vi "background3.vi"() -> ()   [LabVIEW 2014]
uses:
  cloud.ctl
  heart.ctl
  <vilib>/Utility/inputDevices.llb/keyboardAcquire.vi
  <vilib>/Utility/inputDevices.llb/closeKeyboard.vi
panel:
  out "Position:Top 3":i32
  out "Position:Left 3":i32
  out "人1生命":dbl
  out "人2生命":dbl
  out "heart 6":T1
  out "heart 5":T1
  out "heart 4":T1
  out "heart 3":T1
  out "heart 2":T1
  out "heart 1":T1
  out "雲  3":T2
  out "black hole":T3
  out "雲 2":T2
  out "雲":T2
  out "1jump":bool=TRUE
  out "火右飛 2":bool=TRUE
  out "火左飛 2":bool
  out "火左飛":bool
  out "1":T4
  out "火右飛":bool=TRUE
  out "2":T5
  out "2-1":T4
  out "2-2":T5
  in  "stop jump2":bool
  out "Position:Top 2":i32
  out "Position:Left 2":i32
  in  "stop jump1":bool
  out "人1":T6
  out "keys pressed":T7(array[ring])
  in  "right/left 2":bool
  in  "人2":bool
  in  "right/left":bool
  in  "人1":bool
  out "人2":T6
  out "Position:Top":i32
  out "Position:Left":i32
  in  "整個遊戲中止":bool
  # "W:17\nS:31\nA:30\nD:32"
  # "上:72\n下:80\n左:75\n右:77"
  # "17"
  # "48"
  # "587"
  # "168"
  # "523"
  # "623"
  # "678"
  # "334"
  # "288"
  # "408"
  # "1049"
  # "212"
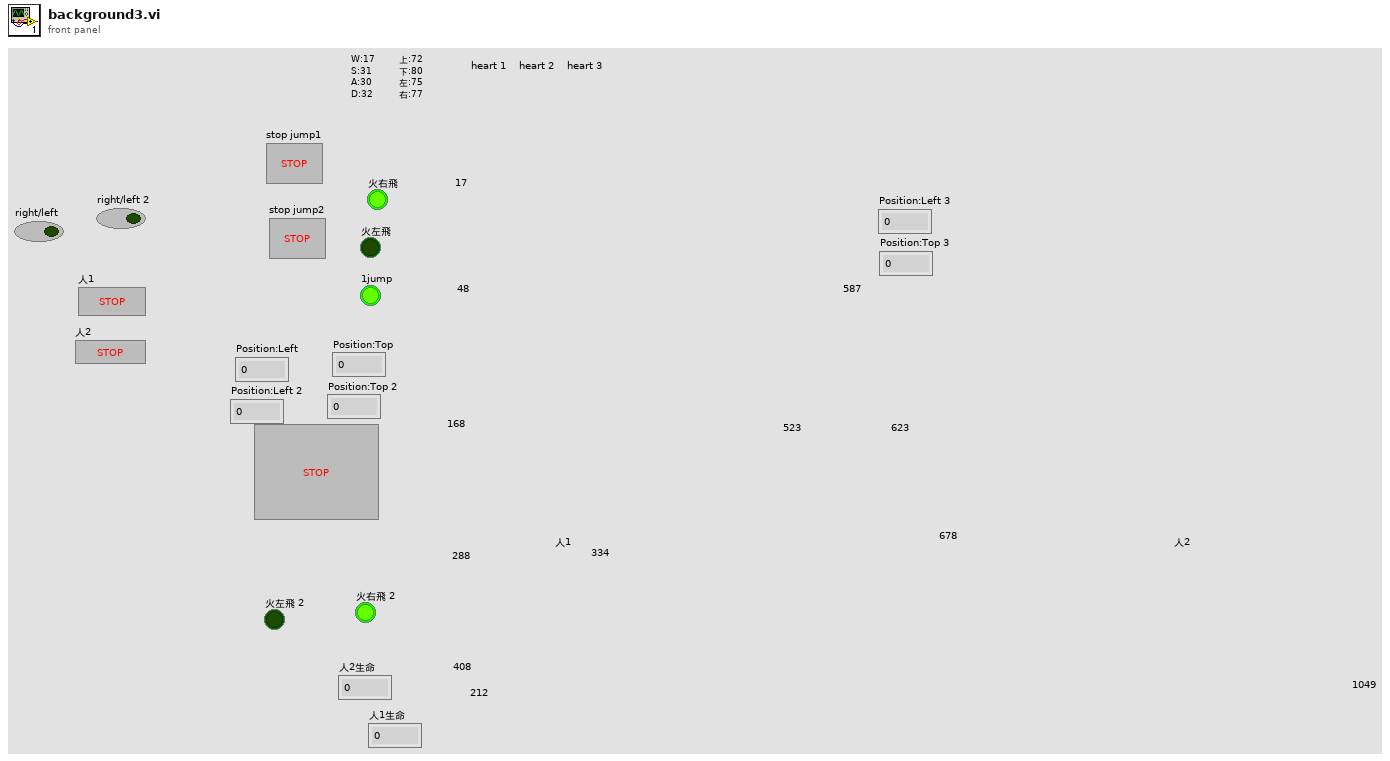
[diagram p1: front panel]
types:
  T1 = typedef "heart.ctl" = u16
  T2 = typedef "cloud.ctl" = u16
  T3 = typedef "Control 4.ctl" = u16
  T4 = typedef "火焰.ctl" = u16
  T5 = typedef "火焰2.ctl" = u16
  T6 = typedef "Control 3.ctl" = u16
  T7 = enum16{"0", "1", "2", "3", "4", "5", "6", "7", "8", "9", "A", "B", "C", "D", "E", "F", "G", "H", "I", "J", "K", "L", "M", "N", "O", "P", "Q", "R", "S", "T", "U", "V", "W", "X", "Y", "Z", "F1", "F2", "F3", "F4", "F5", "F6", "F7", "F8", "F9", "F10", "F11", "F12", "F13", "F14", "F15", "ADD", "BACK", "BACKSLASH", "CAPITAL", "COMMA", "DECIMAL", "DELETE", "DIVIDE", "DOWN", "END", "EQUALS", "ESCAPE", "GRAVE (`)", "HOME", "INSERT", "LBRACKET", "LCONTROL", "LEFT", "L ALT", "LSHIFT", "LWIN", "MINUS", "MULTIPLY", "NEXT", "NUMLOCK", "NUMPAD_0", "NUMPAD_1", "NUMPAD_2", "NUMPAD_3", "NUMPAD_4", "NUMPAD_5", "NUMPAD_6", "NUMPAD_7", "NUMPAD_8", "NUMPAD_9", "PAUSE", "PERIOD", "PRIOR (PG UP)", "RBRACKET", "RCONTROL", "RETURN", "RIGHT", "R ALT", "RSHIFT", "RWIN", "SCROLL", "SEMICOLON", "SLASH", "SPACE", "SUBTRACT", "TAB", "UP", "ENTER (num pad)", "' (quote)"}[]
  T8 = enum16{"0", "1", "2", "3", "4", "5", "6", "7", "8", "9", "A", "B", "C", "D", "E", "F", "G", "H", "I", "J", "K", "L", "M", "N", "O", "P", "Q", "R", "S", "T", "U", "V", "W", "X", "Y", "Z", "F1", "F2", "F3", "F4", "F5", "F6", "F7", "F8", "F9", "F10", "F11", "F12", "F13", "F14", "F15", "ADD", "BACK", "BACKSLASH", "CAPITAL", "COMMA", "DECIMAL", "DELETE", "DIVIDE", "DOWN", "END", "EQUALS", "ESCAPE", "GRAVE (`)", "HOME", "INSERT", "LBRACKET", "LCONTROL", "LEFT", "L ALT", "LSHIFT", "LWIN", "MINUS", "MULTIPLY", "NEXT", "NUMLOCK", "NUMPAD_0", "NUMPAD_1", "NUMPAD_2", "NUMPAD_3", "NUMPAD_4", "NUMPAD_5", "NUMPAD_6", "NUMPAD_7", "NUMPAD_8", "NUMPAD_9", "PAUSE", "PERIOD", "PRIOR (PG UP)", "RBRACKET", "RCONTROL", "RETURN", "RIGHT", "R ALT", "RSHIFT", "RWIN", "SCROLL", "SEMICOLON", "SLASH", "SPACE", "SUBTRACT", "TAB", "UP", "ENTER (num pad)", "' (quote)"}
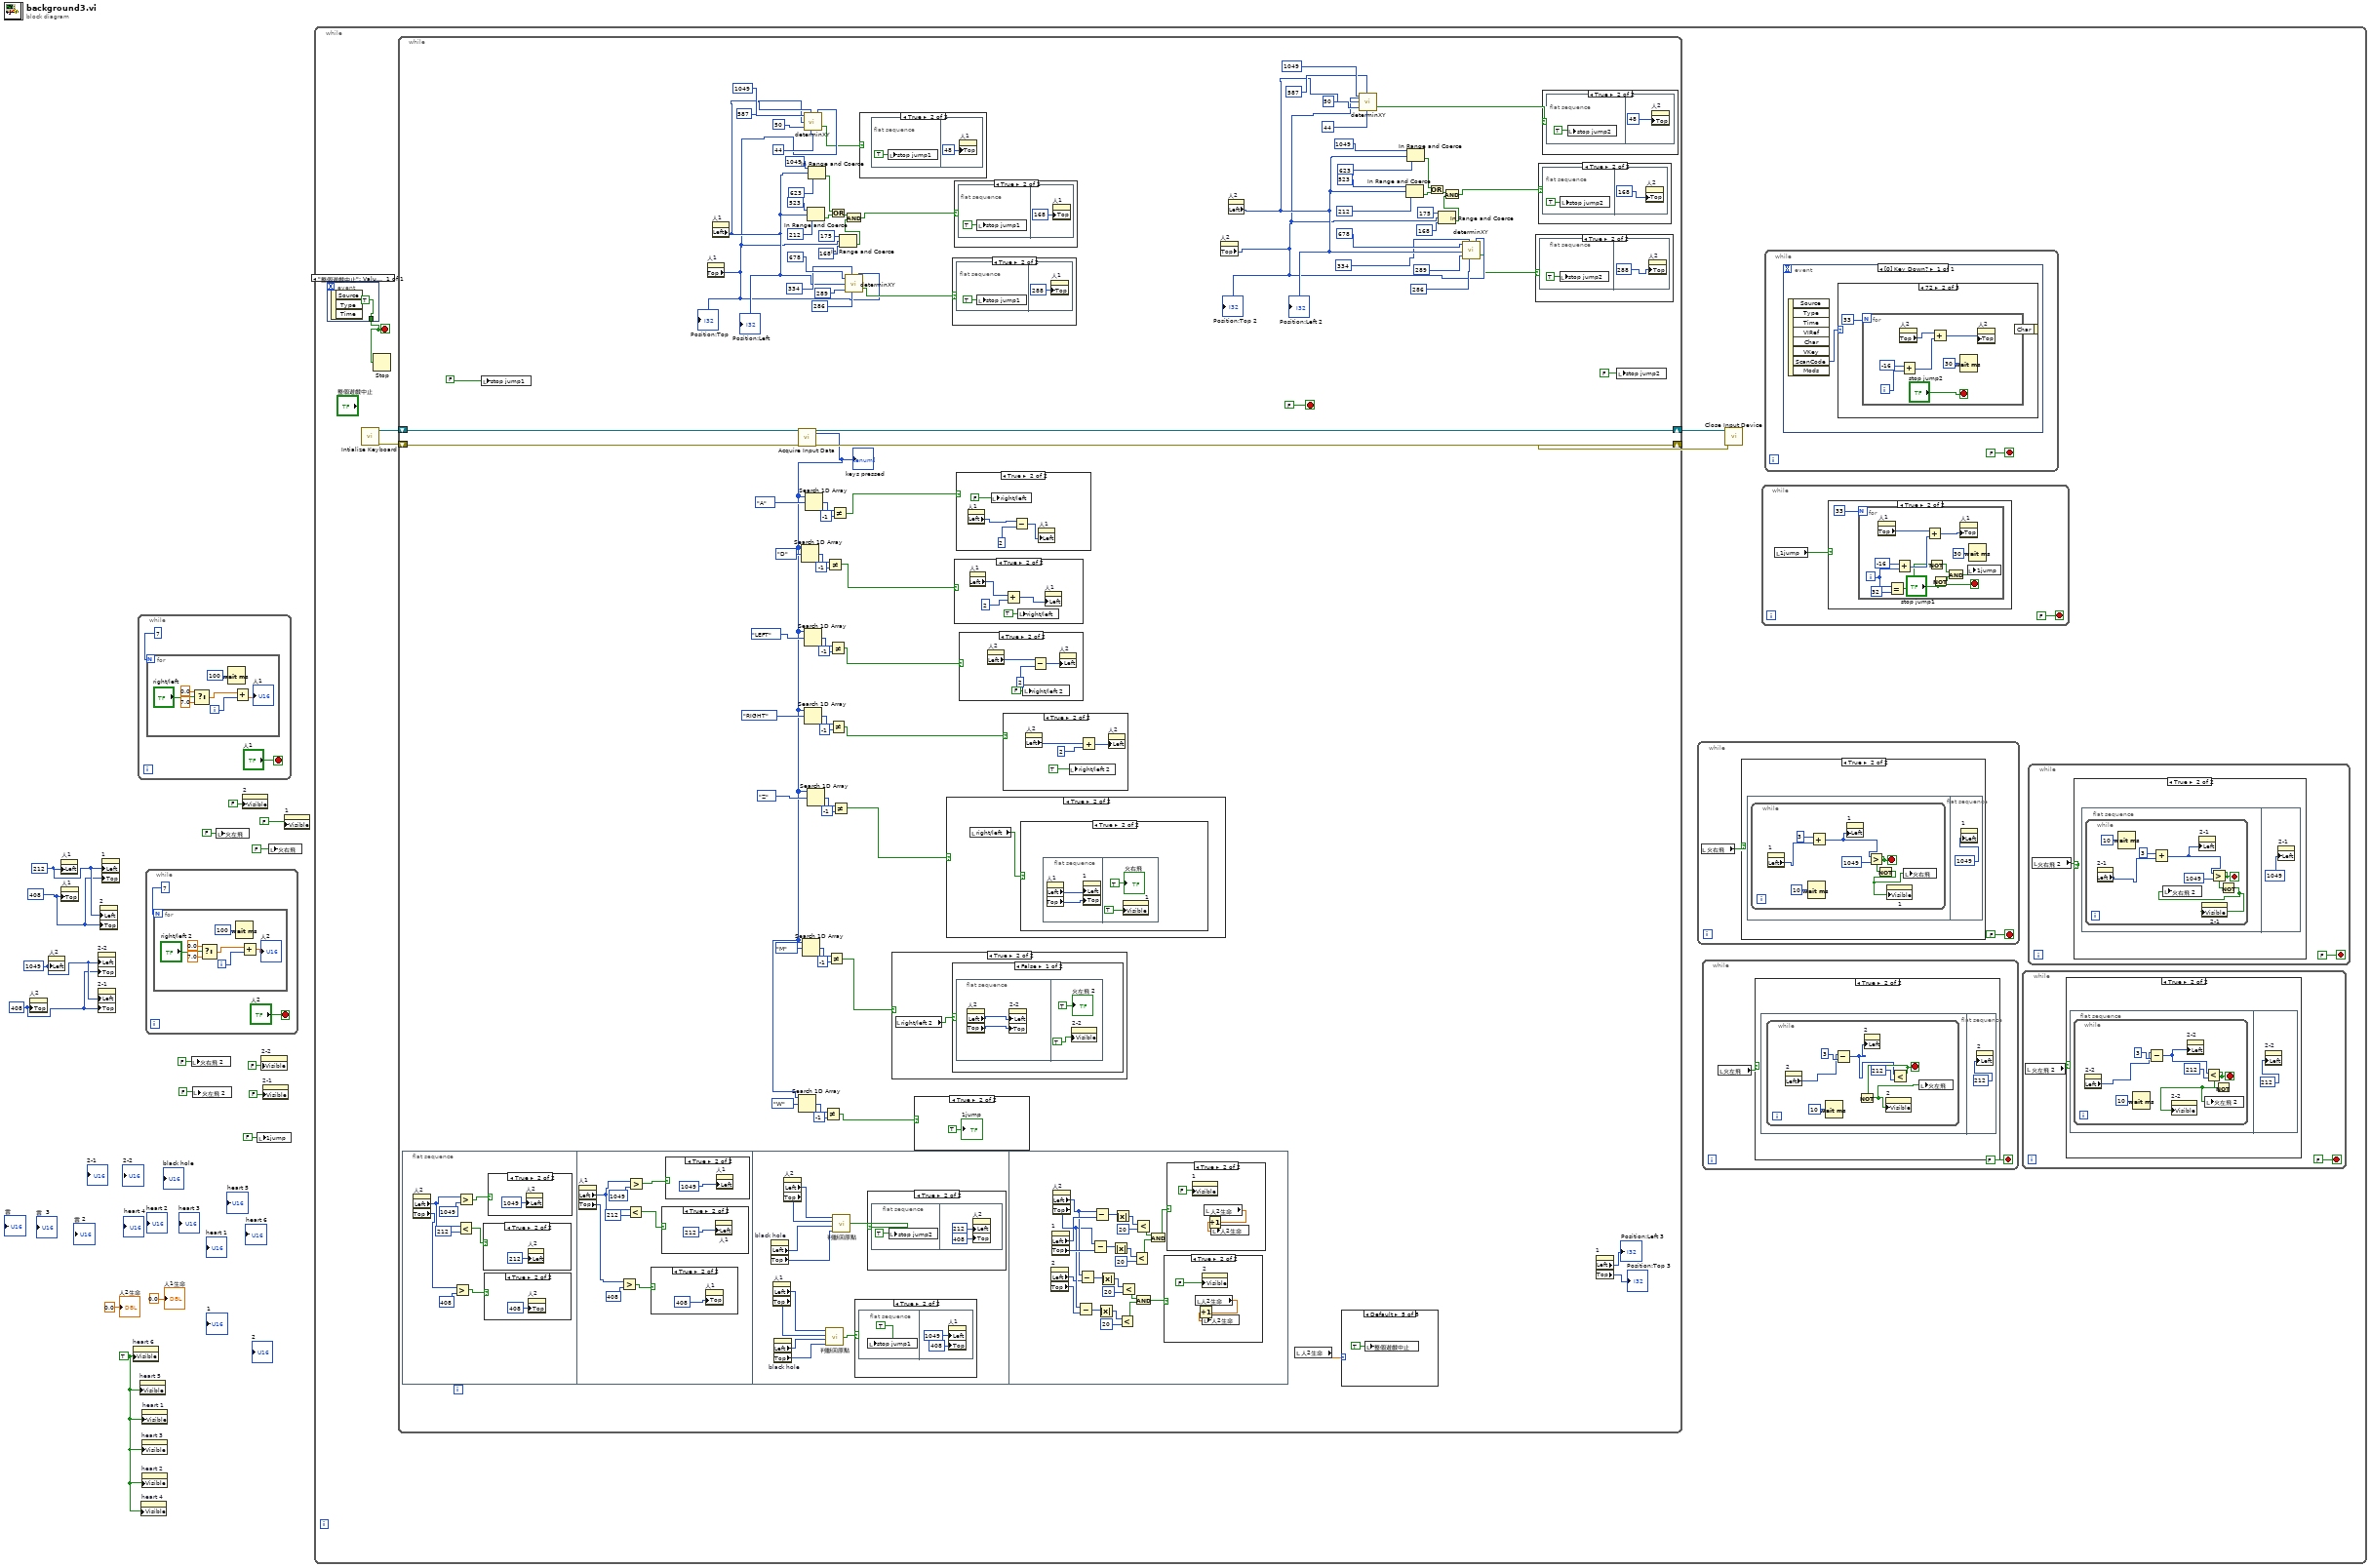
[diagram p0: block diagram]
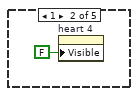
[diagram p10: hidden frame]
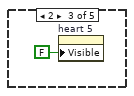
[diagram p11: hidden frame]
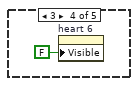
[diagram p12: hidden frame]
diagram:
  w1 = TRUE ("Visible")
  w5 = 408 ("Position:Top")
  w6 = 1049 ("Position:Left")
  w7 = 408 ("Position:Top")
  w8 = 212 ("Position:Left")
  n1 = property on="人2" class="Ring (strict)"("Top"=w5) -> ()  [unwired: 2 in, 2 out]
  n2 = property on="人2" class="Ring (strict)"("Left"=w6) -> ()  [unwired: 2 in, 2 out]
  n3 = property on="人1" class="Ring (strict)"("Left"=w8) -> ()  [unwired: 2 in, 2 out]
  n4 = property on="人1" class="Ring (strict)"("Top"=w7) -> ()  [unwired: 2 in, 2 out]
  n5 = property on="2-2" class="Ring (strict)"("Left"=w6, "Top"=w5) -> ()  [unwired: 2 in, 2 out]
  n6 = property on="2-1" class="Ring (strict)"("Left"=w6, "Top"=w5) -> ()  [unwired: 2 in, 2 out]
  n7 = property on="2" class="Ring (strict)"("Left"=w8, "Top"=w7) -> ()  [unwired: 2 in, 2 out]
  n8 = property on="1" class="Ring (strict)"("Left"=w8, "Top"=w7) -> ()  [unwired: 2 in, 2 out]
  n9 = property on="heart 6" class="Ring (strict)"("Visible"=w1) -> ()  [unwired: 2 in, 2 out]
  n10 = while {
    stop <- "人1" stop-if-true
    n11 = for {
      N: 7 -> [_]
      i -> [w24]
      n12 = Select(t=0.0, s="right/left", f=7.0) -> (s? t:f=w21:dbl)
      n13 = Wait (ms)(milliseconds to wait=u32 100) -> ()  [unwired: 1 out]
      n14 = Add(x=w21, y=w24) -> (x+y=→"人1":dbl)
    }
  }
  n15 = property on="heart 5" class="Ring (strict)"("Visible"=w1) -> ()  [unwired: 2 in, 2 out]
  n16 = property on="heart 4" class="Ring (strict)"("Visible"=w1) -> ()  [unwired: 2 in, 2 out]
  n17 = property on="heart 3" class="Ring (strict)"("Visible"=w1) -> ()  [unwired: 2 in, 2 out]
  n18 = property on="heart 2" class="Ring (strict)"("Visible"=w1) -> ()  [unwired: 2 in, 2 out]
  n19 = property on="heart 1" class="Ring (strict)"("Visible"=w1) -> ()  [unwired: 2 in, 2 out]
  n20 = while {
    stop <- "人2" stop-if-true
    n21 = for {
      N: 7 -> [_]
      i -> [w33]
      n22 = Select(t=0.0, s="right/left 2", f=7.0) -> (s? t:f=w31:dbl)
      n23 = Wait (ms)(milliseconds to wait=u32 100) -> ()  [unwired: 1 out]
      n24 = Add(x=w31, y=w33) -> (x+y=→"人2":dbl)
    }
  }
  n25 = local write "火右飛 2"(FALSE ("火右飛 2")) -> ()
  n26 = local write "火左飛 2"(FALSE ("火左飛 2")) -> ()
  n27 = local write "火左飛"(FALSE ("火左飛")) -> ()
  n28 = property on="2" class="Ring (strict)"("Visible"=FALSE) -> ()  [unwired: 2 in, 2 out]
  n29 = local write "1jump"(FALSE ("1jump")) -> ()
  n30 = property on="2-2" class="Ring (strict)"("Visible"=FALSE) -> ()  [unwired: 2 in, 2 out]
  n31 = property on="2-1" class="Ring (strict)"("Visible"=FALSE) -> ()  [unwired: 2 in, 2 out]
  n32 = local write "火右飛"(FALSE ("Boolean")) -> ()
  n33 = property on="1" class="Ring (strict)"("Visible"=FALSE) -> ()  [unwired: 2 in, 2 out]
  n34 = while {
    stop <- w35 stop-if-true
    n35 = event shown="[0] \"整個遊戲中止\": Value Change" {
      selector: _ -> [_]
      dyn-events: _ -> [_]
      timeout: _ -> [_]
      tunnel: [TRUE] -> w35
      event "整個遊戲中止": Value Change {
        n36 = event-data() -> ()  [unwired: 1 in, 3 out]
      }
    }
    n37 = call <vilib>:"Intialize Keyboard.vi"() -> ("error out"=w38:errorcluster, "device ID"=w39:refnum<k1>)  [unwired: 10 in]
    n38 = Stop(stop? (T)=w35) -> ()
    n39 = while {
      shift-right: [w190] -> w36
      shift-left: w39 -> [w187]
      shift-right: [w189] -> w37
      shift-left: w38 -> [w188]
      stop <- FALSE stop-if-true
      n40 = flat-sequence {
        frame #0 {
          n41 = property on="人2" class="Ring (strict)"() -> ("Left"=w201:i32, "Top"=w196:i32)  [unwired: 2 in, 2 out]
          n42 = Greater?(x=w196, y=408) -> (0:w195:bool)
          n43 = Less?(x=w201, y=212) -> (x < y?=w198:bool)
          n44 = Greater?(x=w201, y=1049) -> (0:w199:bool)
          n45 = case shown="True" w198 {
            frame False {
            }
            frame True {
              n46 = property on="人2" class="Ring (strict)"("Left"=212 ("Position:Left")) -> ()  [unwired: 2 in, 2 out]
            }
          }
          n47 = case shown="True" w195 {
            frame False {
            }
            frame True {
              n48 = property on="人2" class="Ring (strict)"("Top"=408 ("Position:Left")) -> ()  [unwired: 2 in, 2 out]
            }
          }
          n49 = case shown="True" w199 {
            frame False {
            }
            frame True {
              n50 = property on="人2" class="Ring (strict)"("Left"=1049 ("Position:Left")) -> ()  [unwired: 2 in, 2 out]
            }
          }
        }
        frame #1 {
          n51 = property on="人1" class="Ring (strict)"() -> ("Left"=w213:i32, "Top"=w206:i32)  [unwired: 2 in, 2 out]
          n52 = Greater?(x=w206, y=408) -> (0:w208:bool)
          n53 = Less?(x=w213, y=212) -> (x < y?=w212:bool)
          n54 = Greater?(x=w213, y=1049) -> (0:w211:bool)
          n55 = case shown="True" w208 {
            frame False {
            }
            frame True {
              n56 = property on="人1" class="Ring (strict)"("Top"=408 ("Position:Left")) -> ()  [unwired: 2 in, 2 out]
            }
          }
          n57 = case shown="True" w212 {
            frame False {
            }
            frame True {
              n58 = property on="人1" class="Ring (strict)"("Left"=212 ("Position:Left")) -> ()  [unwired: 2 in, 2 out]
            }
          }
          n59 = case shown="True" w211 {
            frame False {
            }
            frame True {
              n60 = property on="人1" class="Ring (strict)"("Left"=1049 ("Position:Left")) -> ()  [unwired: 2 in, 2 out]
            }
          }
        }
        frame #2 {
          n61 = property on="black hole" class="Ring (strict)"() -> ("Left"=w224:i32, "Top"=w223:i32)  [unwired: 2 in, 2 out]
          n62 = property on="人1" class="Ring (strict)"() -> ("Left"=w217:i32, "Top"=w218:i32)  [unwired: 2 in, 2 out]
          n63 = property on="black hole" class="Ring (strict)"() -> ("Left"=w219:i32, "Top"=w220:i32)  [unwired: 2 in, 2 out]
          n64 = property on="人2" class="Ring (strict)"() -> ("Left"=w226:i32, "Top"=w225:i32)  [unwired: 2 in, 2 out]
          n65 = call "判斷回原點.vi"("¬}y"=w220, "¬}x"=w219, "人y"=w218, "人x"=w217) -> ("x .and. y?"=w221:bool)
          n66 = call "判斷回原點.vi"("¬}y"=w223, "¬}x"=w224, "人y"=w225, "人x"=w226) -> ("x .and. y?"=w222:bool)
          n67 = case shown="True" w221 {
            frame False {
            }
            frame True {
              n68 = flat-sequence {
                frame #0 {
                  n69 = local write "stop jump1"(TRUE) -> ()
                }
                frame #1 {
                  n70 = property on="人1" class="Ring (strict)"("Left"=1049 ("Position:Left"), "Top"=408 ("Position:Top")) -> ()  [unwired: 2 in, 2 out]
                }
              }
            }
          }
          n71 = case shown="True" w222 {
            frame False {
            }
            frame True {
              n72 = flat-sequence {
                frame #0 {
                  n73 = local write "stop jump2"(TRUE ("stop jump2")) -> ()
                }
                frame #1 {
                  n74 = property on="人2" class="Ring (strict)"("Left"=212 ("Position:Left"), "Top"=408 ("Position:Top")) -> ()  [unwired: 2 in, 2 out]
                }
              }
            }
          }
        }
        frame #3 {
          n75 = property on="2" class="Ring (strict)"() -> ("Left"=w234:i32, "Top"=w233:i32)  [unwired: 2 in, 2 out]
          n76 = property on="1" class="Ring (strict)"() -> ("Left"=w256:i32, "Top"=w249:i32)  [unwired: 2 in, 2 out]
          n77 = property on="人2" class="Ring (strict)"() -> ("Left"=w236:i32, "Top"=w235:i32)  [unwired: 2 in, 2 out]
          n78 = Subtract(x=w235, y=w233) -> (x-y=w243:i32)
          n79 = Subtract(x=w236, y=w234) -> (x-y=w238:i32)
          n80 = Subtract(x=w235, y=w249) -> (x-y=w250:i32)
          n81 = Subtract(x=w236, y=w256) -> (x-y=w255:i32)
          n82 = Absolute Value(x=w243) -> (abs(x)=w242:i32)
          n83 = Absolute Value(x=w238) -> (abs(x)=w239:i32)
          n84 = Absolute Value(x=w250) -> (abs(x)=w251:i32)
          n85 = Absolute Value(x=w255) -> (abs(x)=w254:i32)
          n86 = Less?(x=w242, y=20) -> (x < y?=w245:bool)
          n87 = Less?(x=w239, y=20) -> (x < y?=w244:bool)
          n88 = Less?(x=w251, y=20) -> (x < y?=w247:bool)
          n89 = Less?(x=w254, y=20) -> (x < y?=w248:bool)
          n90 = And(x=w244, y=w245) -> (x .and. y?=w237:bool)
          n91 = And(x=w248, y=w247) -> (x .and. y?=w246:bool)
          n92 = case shown="True" w237 {
            frame False {
            }
            frame True {
              n93 = local read "人2生命"() -> (w257:dbl)
              n94 = Increment(x=w257) -> (x+1=w258:dbl)
              n95 = property on="2" class="Ring (strict)"("Visible"=FALSE) -> ()  [unwired: 2 in, 2 out]
              n96 = local write "人2生命"(w258) -> ()
            }
          }
          n97 = case shown="True" w246 {
            frame False {
            }
            frame True {
              n98 = property on="1" class="Ring (strict)"("Visible"=FALSE) -> ()  [unwired: 2 in, 2 out]
              n99 = local read "人2生命"() -> (w261:dbl)
              n100 = Increment(x=w261) -> (x+1=w260:dbl)
              n101 = local write "人2生命"(w260) -> ()
            }
          }
        }
      }
      n102 = local write "stop jump1"(FALSE ("stop jump1")) -> ()
      n103 = property on="人1" class="Ring (strict)"() -> ("Top"=w122:i32)  [unwired: 2 in, 2 out]
      "Position:Top" <- w122
      n104 = property on="人1" class="Ring (strict)"() -> ("Left"=w125:i32)  [unwired: 2 in, 2 out]
      "Position:Left" <- w125
      n105 = call-poly <vilib>:"Acquire Input Data.vi"("device ID"=w187, "error in (no error)"=w188) -> ("device ID"=w190:refnum<k1>, "keys pressed"=w134:T7, "error out"=w189:errorcluster)  [unwired: 15 in]
      "keys pressed" <- w134
      n106 = Search 1D Array(1D array=w134, element=T8."W") -> (index of element=w136:i32)  [unwired: 1 in]
      n107 = Search 1D Array(1D array=w134, element=T8."D") -> (index of element=w181:i32)  [unwired: 1 in]
      n108 = Search 1D Array(1D array=w134, element=T8."M") -> (index of element=w143:i32)  [unwired: 1 in]
      n109 = call "determinXY.vi"("x max"=1049 ("upper limit"), "x min"=587 ("lower limit"), "x"=w125, "y max"=50 ("upper limit"), "y min"=44 ("lower limit"), "y"=w122) -> ("result"=w121:bool)
      n110 = Search 1D Array(1D array=w134, element=T8."LEFT") -> (index of element=w178:i32)  [unwired: 1 in]
      n111 = Search 1D Array(1D array=w134, element=T8."RIGHT") -> (index of element=w174:i32)  [unwired: 1 in]
      n112 = Search 1D Array(1D array=w134, element=T8."A") -> (index of element=w184:i32)  [unwired: 1 in]
      n113 = Search 1D Array(1D array=w134, element=T8."Z") -> (index of element=w146:i32)  [unwired: 1 in]
      n114 = In Range and Coerce(upper limit=523, x=w125, lower limit=212) -> (In Range?=w161:bool)  [unwired: 1 out]
      n115 = In Range and Coerce(upper limit=1049, x=w125, lower limit=623) -> (In Range?=w162:bool)  [unwired: 1 out]
      n116 = Not Equal?(x=w136, y=-1) -> (x != y?=w133:bool)
      n117 = Not Equal?(x=w181, y=-1) -> (x != y?=w139:bool)
      n118 = Not Equal?(x=w143, y=-1) -> (x != y?=w141:bool)
      n119 = Not Equal?(x=w178, y=-1) -> (x != y?=w176:bool)
      n120 = Or(x=w162, y=w161) -> (x .or. y?=w163:bool)
      n121 = Not Equal?(x=w174, y=-1) -> (x != y?=w172:bool)
      n122 = Not Equal?(x=w184, y=-1) -> (x != y?=w140:bool)
      n123 = Not Equal?(x=w146, y=-1) -> (x != y?=w138:bool)
      n124 = In Range and Coerce(upper limit=175, x=w122, lower limit=168 ("y")) -> (In Range?=w167:bool)  [unwired: 1 out]
      n125 = And(x=w163, y=w167) -> (x .and. y?=w160:bool)
      n126 = call "determinXY.vi"("x max"=678 ("upper limit"), "x min"=334 ("lower limit"), "x"=w125, "y max"=289 ("upper limit"), "y min"=286 ("y"), "y"=w122) -> ("result"=w128:bool)
      n127 = case shown="True" w121 {
        frame False {
        }
        frame True {
          n128 = flat-sequence {
            frame #0 {
              n129 = local write "stop jump1"(TRUE ("stop jump1")) -> ()
            }
            frame #1 {
              n130 = property on="人1" class="Ring (strict)"("Top"=48 ("Position:Top")) -> ()  [unwired: 2 in, 2 out]
            }
          }
        }
      }
      n131 = case shown="True" w141 {
        frame False {
        }
        frame True {
          n132 = local read "right/left 2"() -> (w264:bool)
          n133 = case shown="False" w264 {
            frame False {
              n134 = flat-sequence {
                frame #0 {
                  n135 = property on="人2" class="Ring (strict)"() -> ("Left"=w266:i32, "Top"=w265:i32)  [unwired: 2 in, 2 out]
                  n136 = property on="2-2" class="Ring (strict)"("Left"=w266, "Top"=w265) -> ()  [unwired: 2 in, 2 out]
                }
                frame #1 {
                  n137 = property on="2-2" class="Ring (strict)"("Visible"=TRUE) -> ()  [unwired: 2 in, 2 out]
                  "火左飛 2" <- TRUE
                }
              }
            }
            frame True {
              n138 = flat-sequence {
                frame #0 {
                  n139 = property on="人2" class="Ring (strict)"() -> ("Left"=w270:i32, "Top"=w269:i32)  [unwired: 2 in, 2 out]
                  n140 = property on="2-1" class="Ring (strict)"("Left"=w270, "Top"=w269) -> ()  [unwired: 2 in, 2 out]
                }
                frame #1 {
                  n141 = property on="2-1" class="Ring (strict)"("Visible"=TRUE) -> ()  [unwired: 2 in, 2 out]
                  "火右飛 2" <- TRUE
                }
              }
            }
          }
        }
      }
      n142 = case shown="True" w133 {
        frame False {
        }
        frame True {
          "1jump" <- TRUE
        }
      }
      n143 = case shown="True" w138 {
        frame False {
        }
        frame True {
          n144 = local read "right/left"() -> (w273:bool)
          n145 = case shown="True" w273 {
            frame False {
              n146 = flat-sequence {
                frame #0 {
                  n147 = property on="人1" class="Ring (strict)"() -> ("Left"=w275:i32, "Top"=w274:i32)  [unwired: 2 in, 2 out]
                  n148 = property on="2" class="Ring (strict)"("Left"=w275, "Top"=w274) -> ()  [unwired: 2 in, 2 out]
                }
                frame #1 {
                  n149 = property on="2" class="Ring (strict)"("Visible"=TRUE) -> ()  [unwired: 2 in, 2 out]
                  "火左飛" <- TRUE
                }
              }
            }
            frame True {
              n150 = flat-sequence {
                frame #0 {
                  n151 = property on="人1" class="Ring (strict)"() -> ("Left"=w279:i32, "Top"=w278:i32)  [unwired: 2 in, 2 out]
                  n152 = property on="1" class="Ring (strict)"("Left"=w279, "Top"=w278) -> ()  [unwired: 2 in, 2 out]
                }
                frame #1 {
                  n153 = property on="1" class="Ring (strict)"("Visible"=TRUE) -> ()  [unwired: 2 in, 2 out]
                  "火右飛" <- TRUE
                }
              }
            }
          }
        }
      }
      n154 = case shown="True" w128 {
        frame False {
        }
        frame True {
          n155 = flat-sequence {
            frame #0 {
              n156 = local write "stop jump1"(TRUE ("stop jump1")) -> ()
            }
            frame #1 {
              n157 = property on="人1" class="Ring (strict)"("Top"=288 ("Position:Top")) -> ()  [unwired: 2 in, 2 out]
            }
          }
        }
      }
      n158 = case shown="True" w160 {
        frame False {
        }
        frame True {
          n159 = flat-sequence {
            frame #0 {
              n160 = local write "stop jump1"(TRUE ("stop jump1")) -> ()
            }
            frame #1 {
              n161 = property on="人1" class="Ring (strict)"("Top"=168 ("Position:Top")) -> ()  [unwired: 2 in, 2 out]
            }
          }
        }
      }
      n162 = case shown="True" w139 {
        frame False {
        }
        frame True {
          n163 = property on="人1" class="Ring (strict)"() -> ("Left"=w304:i32)  [unwired: 2 in, 2 out]
          n164 = Add(x=w304, y=2) -> (x+y=w303:i32)
          n165 = local write "right/left"(TRUE ("right/left")) -> ()
          n166 = property on="人1" class="Ring (strict)"("Left"=w303) -> ()  [unwired: 2 in, 2 out]
        }
      }
      n167 = case shown="True" w140 {
        frame False {
        }
        frame True {
          n168 = property on="人1" class="Ring (strict)"() -> ("Left"=w307:i32)  [unwired: 2 in, 2 out]
          n169 = local write "right/left"(FALSE ("人1 right 2")) -> ()
          n170 = Subtract(x=w307, y=2) -> (x-y=w306:i32)
          n171 = property on="人1" class="Ring (strict)"("Left"=w306) -> ()  [unwired: 2 in, 2 out]
        }
      }
      n172 = case shown="True" w176 {
        frame False {
        }
        frame True {
          n173 = property on="人2" class="Ring (strict)"() -> ("Left"=w300:i32)  [unwired: 2 in, 2 out]
          n174 = local write "right/left 2"(FALSE ("right/left")) -> ()
          n175 = Subtract(x=w300, y=2) -> (x-y=w299:i32)
          n176 = property on="人2" class="Ring (strict)"("Left"=w299) -> ()  [unwired: 2 in, 2 out]
        }
      }
      n177 = case shown="True" w172 {
        frame False {
        }
        frame True {
          n178 = property on="人2" class="Ring (strict)"() -> ("Left"=w296:i32)  [unwired: 2 in, 2 out]
          n179 = local write "right/left 2"(TRUE ("人1 right 2")) -> ()
          n180 = Add(x=w296, y=2) -> (x+y=w295:i32)
          n181 = property on="人2" class="Ring (strict)"("Left"=w295) -> ()  [unwired: 2 in, 2 out]
        }
      }
      n182 = property on="人2" class="Ring (strict)"() -> ("Top"=w110:i32)  [unwired: 2 in, 2 out]
      "Position:Top 2" <- w110
      n183 = property on="人2" class="Ring (strict)"() -> ("Left"=w114:i32)  [unwired: 2 in, 2 out]
      "Position:Left 2" <- w114
      n184 = local read "人2生命"() -> (w106:dbl)
      n185 = case shown="Default" w106 {
        frame 0 {
        }
        frame 1 {
          n186 = property on="heart 4" class="Ring (strict)"("Visible"=FALSE) -> ()  [unwired: 2 in, 2 out]
        }
        frame 2 {
          n187 = property on="heart 5" class="Ring (strict)"("Visible"=FALSE) -> ()  [unwired: 2 in, 2 out]
        }
        frame 3 {
          n188 = property on="heart 6" class="Ring (strict)"("Visible"=FALSE) -> ()  [unwired: 2 in, 2 out]
        }
        frame Default {
          n189 = local write "整個遊戲中止"(TRUE ("整個遊戲中止")) -> ()
        }
      }
      n190 = call "determinXY.vi"("x max"=1049 ("upper limit"), "x min"=587 ("lower limit"), "x"=w114, "y max"=50 ("upper limit"), "y min"=44 ("lower limit"), "y"=w110) -> ("result"=w116:bool)
      n191 = In Range and Coerce(upper limit=523, x=w114, lower limit=212) -> (In Range?=w150:bool)  [unwired: 1 out]
      n192 = In Range and Coerce(upper limit=1049, x=w114, lower limit=623) -> (In Range?=w151:bool)  [unwired: 1 out]
      n193 = Or(x=w151, y=w150) -> (x .or. y?=w152:bool)
      n194 = In Range and Coerce(upper limit=175, x=w110, lower limit=168 ("y")) -> (In Range?=w155:bool)  [unwired: 1 out]
      n195 = And(x=w152, y=w155) -> (x .and. y?=w149:bool)
      n196 = call "determinXY.vi"("x max"=678 ("upper limit"), "x min"=334 ("lower limit"), "x"=w114, "y max"=289 ("upper limit"), "y min"=286 ("y"), "y"=w110) -> ("result"=w109:bool)
      n197 = case shown="True" w109 {
        frame False {
        }
        frame True {
          n198 = flat-sequence {
            frame #0 {
              n199 = local write "stop jump2"(TRUE ("stop jump1")) -> ()
            }
            frame #1 {
              n200 = property on="人2" class="Ring (strict)"("Top"=288 ("Position:Top")) -> ()  [unwired: 2 in, 2 out]
            }
          }
        }
      }
      n201 = case shown="True" w149 {
        frame False {
        }
        frame True {
          n202 = flat-sequence {
            frame #0 {
              n203 = local write "stop jump2"(TRUE ("stop jump1")) -> ()
            }
            frame #1 {
              n204 = property on="人2" class="Ring (strict)"("Top"=168 ("Position:Top")) -> ()  [unwired: 2 in, 2 out]
            }
          }
        }
      }
      n205 = case shown="True" w116 {
        frame False {
        }
        frame True {
          n206 = flat-sequence {
            frame #0 {
              n207 = local write "stop jump2"(TRUE ("stop jump1")) -> ()
            }
            frame #1 {
              n208 = property on="人2" class="Ring (strict)"("Top"=48 ("Position:Top")) -> ()  [unwired: 2 in, 2 out]
            }
          }
        }
      }
      n209 = property on="1" class="Ring (strict)"() -> ("Left"=→"Position:Left 3":i32, "Top"=→"Position:Top 3":i32)  [unwired: 2 in, 2 out]
      n210 = local write "stop jump2"(FALSE ("stop jump1 2")) -> ()
    }
    n211 = while {
      stop <- FALSE stop-if-true
      n212 = local read "火右飛"() -> (w77:bool)
      n213 = case shown="True" w77 {
        frame False {
        }
        frame True {
          n214 = flat-sequence {
            frame #0 {
              n215 = while {
                stop <- w82 stop-if-true
                n216 = property on="1" class="Ring (strict)"() -> ("Left"=w81:i32)  [unwired: 2 in, 2 out]
                n217 = Wait (ms)(milliseconds to wait=u32 10) -> ()  [unwired: 1 out]
                n218 = Add(x=3, y=w81) -> (x+y=w80:i32)
                n219 = property on="1" class="Ring (strict)"("Left"=w80) -> ()  [unwired: 2 in, 2 out]
                n220 = Greater?(x=w80, y=1049) -> (0:w82:bool)
                n221 = Not(x=w82) -> (.not. x?=w78:bool)
                n222 = property on="1" class="Ring (strict)"("Visible"=w78) -> ()  [unwired: 2 in, 2 out]
                n223 = local write "火右飛"(w78) -> ()
              }
            }
            frame #1 {
              n224 = property on="1" class="Ring (strict)"("Left"=1049 ("y")) -> ()  [unwired: 2 in, 2 out]
            }
          }
        }
      }
    }
    n225 = while {
      stop <- FALSE stop-if-true
      n226 = local read "火左飛"() -> (w87:bool)
      n227 = case shown="True" w87 {
        frame False {
        }
        frame True {
          n228 = flat-sequence {
            frame #0 {
              n229 = while {
                stop <- w94 stop-if-true
                n230 = property on="2" class="Ring (strict)"() -> ("Left"=w92:i32)  [unwired: 2 in, 2 out]
                n231 = Wait (ms)(milliseconds to wait=u32 10) -> ()  [unwired: 1 out]
                n232 = Subtract(x=w92, y=3 ("x")) -> (x-y=w89:i32)
                n233 = property on="2" class="Ring (strict)"("Left"=w89) -> ()  [unwired: 2 in, 2 out]
                n234 = Less?(x=w89, y=212) -> (x < y?=w94:bool)
                n235 = Not(x=w94) -> (.not. x?=w88:bool)
                n236 = property on="2" class="Ring (strict)"("Visible"=w88) -> ()  [unwired: 2 in, 2 out]
                n237 = local write "火左飛"(w88) -> ()
              }
            }
            frame #1 {
              n238 = property on="2" class="Ring (strict)"("Left"=212 ("y")) -> ()  [unwired: 2 in, 2 out]
            }
          }
        }
      }
    }
    n239 = call-poly <vilib>:"Close Input Device.vi"("error in (no error)"=w37, "device ID"=w36) -> ()  [unwired: 8 in, 1 out]
    n240 = while {
      stop <- FALSE stop-if-true
      n241 = local read "1jump"() -> (w41:bool)
      n242 = case shown="True" w41 {
        frame False {
        }
        frame True {
          n243 = for {
            N: 33 -> [_]
            i -> [w49]
            stop <- "stop jump1" stop-if-true
            n244 = property on="人1" class="Ring (strict)"() -> ("Top"=w52:i32)  [unwired: 2 in, 2 out]
            n245 = Equal?(x=w49, y=32) -> (x = y?=w47:bool)
            n246 = Add(x=-16, y=w49) -> (x+y=w54:i32)
            n247 = Add(x=w52, y=w54) -> (x+y=w51:i32)
            n248 = Not(x=w47) -> (.not. x?=w46:bool)
            n249 = Not(x="stop jump1") -> (.not. x?=w45:bool)
            n250 = And(x=w46, y=w45) -> (x .and. y?=w44:bool)
            n251 = property on="人1" class="Ring (strict)"("Top"=w51) -> ()  [unwired: 2 in, 2 out]
            n252 = local write "1jump"(w44) -> ()
            n253 = Wait (ms)(milliseconds to wait=u32 30) -> ()  [unwired: 1 out]
          }
        }
      }
    }
    n254 = while {
      stop <- FALSE stop-if-true
      n255 = event shown="[0] Key Down?" {
        selector: _ -> [_]
        dyn-events: _ -> [_]
        timeout: _ -> [_]
        event Key Down? {
          n256 = event-data() -> ("ScanCode"=w97:i16)  [unwired: 1 in, 7 out]
          n257 = case shown="72" w97 {
            frame Default {
            }
            frame 72 {
              n258 = for {
                N: 33 -> [_]
                i -> [w105]
                stop <- "stop jump2" stop-if-true
                n259 = property on="人2" class="Ring (strict)"() -> ("Top"=w101:i32)  [unwired: 2 in, 2 out]
                n260 = Add(x=-16, y=w105) -> (x+y=w103:i32)
                n261 = Add(x=w101, y=w103) -> (x+y=w100:i32)
                n262 = Wait (ms)(milliseconds to wait=u32 30) -> ()  [unwired: 1 out]
                n263 = property on="人2" class="Ring (strict)"("Top"=w100) -> ()  [unwired: 2 in, 2 out]
              }
            }
            frame 17 {
            }
          }
          n264 = event-data() -> ()  [unwired: 2 in, 1 out]
        }
      }
    }
    n265 = while {
      stop <- FALSE stop-if-true
      n266 = local read "火左飛 2"() -> (w57:bool)
      n267 = case shown="True" w57 {
        frame False {
        }
        frame True {
          n268 = flat-sequence {
            frame #0 {
              n269 = while {
                stop <- w64 stop-if-true
                n270 = property on="2-2" class="Ring (strict)"() -> ("Left"=w62:i32)  [unwired: 2 in, 2 out]
                n271 = Wait (ms)(milliseconds to wait=u32 10) -> ()  [unwired: 1 out]
                n272 = Subtract(x=w62, y=3 ("x")) -> (x-y=w59:i32)
                n273 = property on="2-2" class="Ring (strict)"("Left"=w59) -> ()  [unwired: 2 in, 2 out]
                n274 = Less?(x=w59, y=212) -> (x < y?=w64:bool)
                n275 = Not(x=w64) -> (.not. x?=w58:bool)
                n276 = property on="2-2" class="Ring (strict)"("Visible"=w58) -> ()  [unwired: 2 in, 2 out]
                n277 = local write "火左飛 2"(w58) -> ()
              }
            }
            frame #1 {
              n278 = property on="2-2" class="Ring (strict)"("Left"=212 ("y")) -> ()  [unwired: 2 in, 2 out]
            }
          }
        }
      }
    }
    n279 = while {
      stop <- FALSE stop-if-true
      n280 = local read "火右飛 2"() -> (w67:bool)
      n281 = case shown="True" w67 {
        frame False {
        }
        frame True {
          n282 = flat-sequence {
            frame #0 {
              n283 = while {
                stop <- w72 stop-if-true
                n284 = property on="2-1" class="Ring (strict)"() -> ("Left"=w71:i32)  [unwired: 2 in, 2 out]
                n285 = Wait (ms)(milliseconds to wait=u32 10) -> ()  [unwired: 1 out]
                n286 = Add(x=3, y=w71) -> (x+y=w70:i32)
                n287 = property on="2-1" class="Ring (strict)"("Left"=w70) -> ()  [unwired: 2 in, 2 out]
                n288 = Greater?(x=w70, y=1049) -> (0:w72:bool)
                n289 = Not(x=w72) -> (.not. x?=w68:bool)
                n290 = local write "火右飛 2"(w68) -> ()
                n291 = property on="2-1" class="Ring (strict)"("Visible"=w68) -> ()  [unwired: 2 in, 2 out]
              }
            }
            frame #1 {
              n292 = property on="2-1" class="Ring (strict)"("Left"=1049 ("y")) -> ()  [unwired: 2 in, 2 out]
            }
          }
        }
      }
    }
  }
  "人2生命" <- 0.0 ("人1生命")
  "人1生命" <- 0.0 ("人2生命")
